vi "Calculate RO using SensorDAQ.vi"() -> ()   [LabVIEW 2012]
uses:
  <vilib>/Utility/file.llb/Write To Spreadsheet File (string).vi
panel:
  out "Elapsed Time (s)":dbl
  in  "file path (use dialog)":path
  out "MQ9 and MQ131 Raw Voltage Levels":T1(graph)
  out "AI1 MQ131 Ozone Sensor":dbl caption="AI1 pin 12 RSE"
  out "AI0 MQ9 Gas Sensor":dbl caption="AI0 pin 11 RSE"
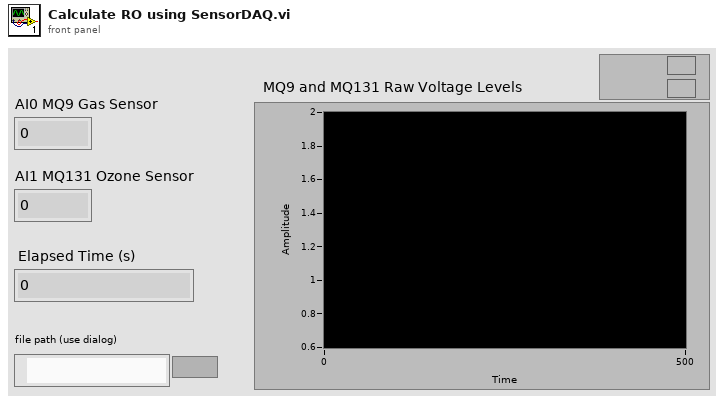
[diagram p1: front panel]
types:
  T1 = cluster{"AI0 pin 11 RSE ":dbl, "AI1 pin 12 RSE ":dbl}
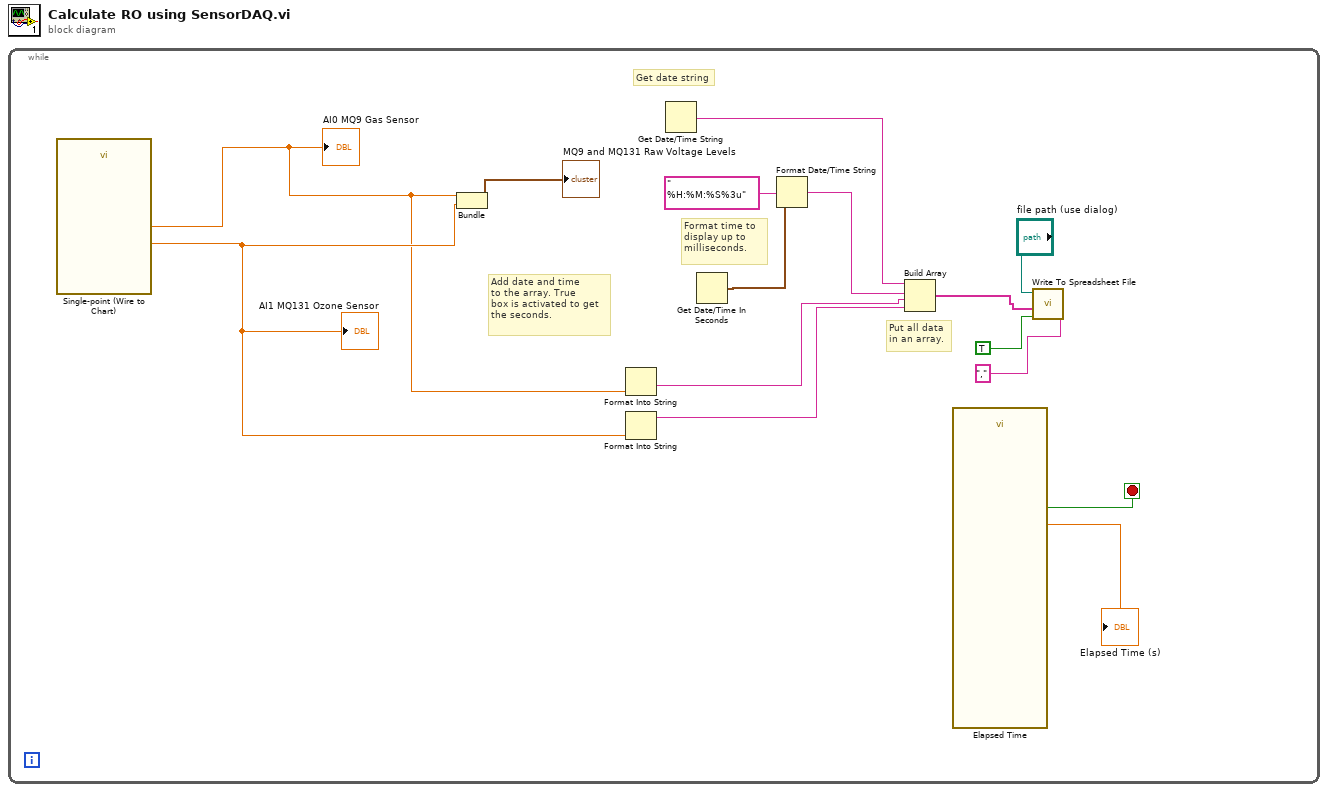
[diagram p0: block diagram]
diagram:
  n1 = while {
    stop <- w3 stop-if-true
    # "Put all data\nin an array."
    # "Format time to \ndisplay up to\nmilliseconds."
    # "Get date string"
    # "Add date and time\nto the array. True \nbox is activated to get \nthe seconds."
    n2 = call "Single-point (Wire to Chart)"() -> ("AI0 pin 11 RSE"=w2:dbl, "AI1 pin 12 RSE"=w11:dbl)  [unwired: 15 in, 3 out]
    "AI0 MQ9 Gas Sensor" <- w2
    "AI1 MQ131 Ozone Sensor" <- w11
    n3 = Bundle("AI0 pin 11 RSE"=w2, "AI1 pin 12 RSE"=w11) -> (→"MQ9 and MQ131 Raw Voltage Levels":T1)  [unwired: 1 in]
    n4 = Format Into String(w2) -> (resulting string=w5:string)  [unwired: 3 in, 1 out]
    n5 = Format Into String(w11) -> (resulting string=w4:string)  [unwired: 3 in, 1 out]
    n6 = Get Date/Time String() -> (date string=w9:string)  [unwired: 3 in, 1 out]
    n7 = Get Date/Time In Seconds() -> (seconds since 1Jan1904=w7:timestamp)
    n8 = Format Date/Time String(time format string (%c)="            %H:%M:%S%3u", seconds (now)=w7) -> (date/time string=w8:string)  [unwired: 1 in]
    n9 = Build Array(w9, w8, w5, w4) -> (w6:string[])
    n10 = call "Elapsed Time"() -> ("Elapsed Time (s)"=→"Elapsed Time (s)":dbl, "Time has Elapsed"=w3:bool)  [unwired: 12 in, 6 out]
    n11 = call-poly <vilib>:"Write To Spreadsheet File.vi"("delimiter (\\t)"="," ("delimiter (\\t)"), "append to file? (new file:F)"=TRUE, "1D data"=w6, "file path (dialog if empty)"="file path (use dialog)") -> ()  [unwired: 4 in, 1 out]
  }
